vi "StringifiedData.vi"(8 "error in (no error)":errorcluster, 11 "BooleanMsg in":refnum<class "BooleanMsg.lvclass">) -> (0 "error out":errorcluster, 2 "Stringified Data":string, 3 "BooleanMsg out":refnum<class "BooleanMsg.lvclass">)   [LabVIEW 2017, in "LapDog.Messaging.v3.NativeTypes.lvlib" / "BooleanMsg.lvclass"]
doc: "This VI is used for the message probe. Child classes may override it and provide the message data in string format or a short string describing the data the message contains. This string will be displayed in the probe window."
uses:
  BooleanMsg.lvclass
  BooleanMsg.lvclass/BooleanMsg.ctl
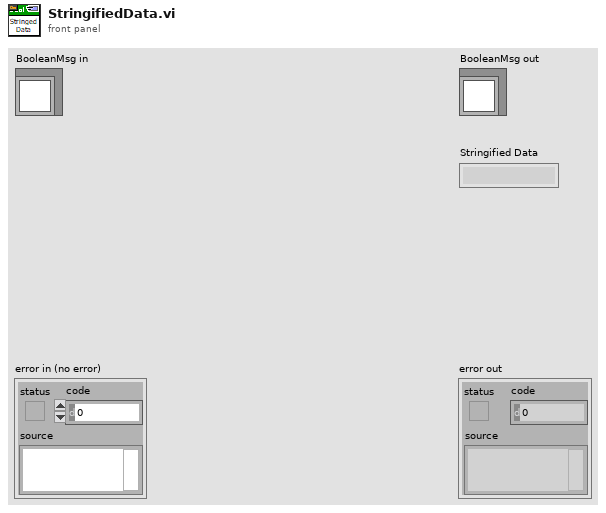
[diagram p1: front panel]
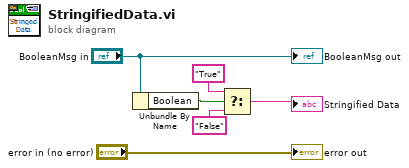
[diagram p0: block diagram]
diagram:
  n1 = Unbundle By Name("BooleanMsg in") -> ("Boolean"=w4:bool)
  n2 = Select(t="True", s=w4, f="False") -> (s? t:f=→"Stringified Data":string)
  "error out" <- "error in (no error)"
  "BooleanMsg out" <- "BooleanMsg in"
